vi "Cabecera.vi"() -> (0 "String":string)   [LabVIEW 2015]
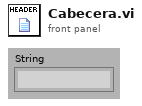
[diagram p1: front panel]
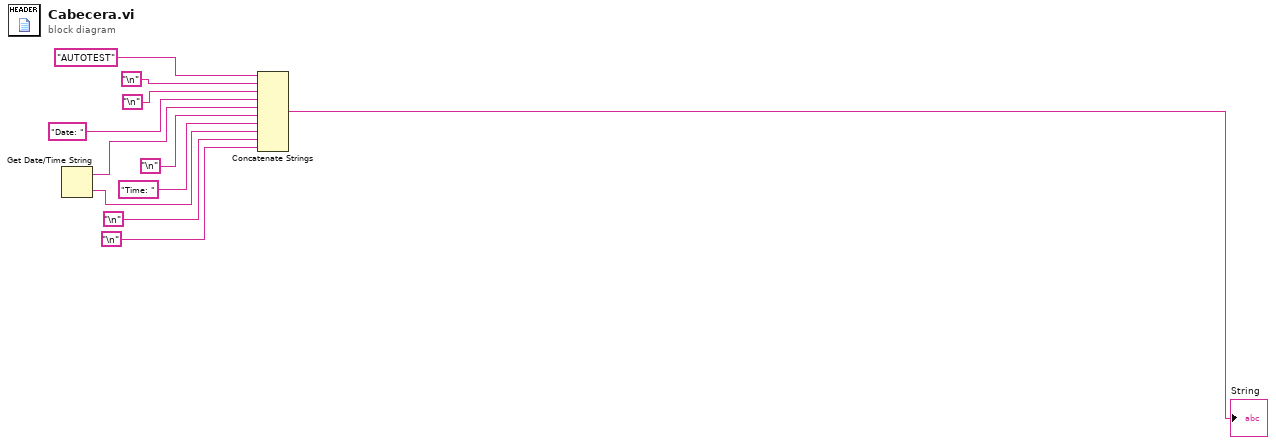
[diagram p0: block diagram]
diagram:
  n1 = Get Date/Time String() -> (date string=w5:string, time string=w8:string)  [unwired: 3 out]
  n2 = Concatenate Strings("AUTOTEST", "\n", "\n", "Date: ", w5, "\n", "Time: ", w8, "\n", "\n") -> (→"String":string)
